vi "SubVI_PupilDetection_COLSxROWS.vi"(0 "arr":u8[][](array[numeric]), 1 "AT":u8, 2 "GB":u8, 3 "N_pts":u8, 4 "img_rows":u16=1024, 5 "img_cols":u16=1280) -> (14 "Pup_x":i16, 15 "Pup_y":i16, 16 "Radius":i16, 17 "Radius_STD":i16, 19 "error out":errorcluster)   [LabVIEW 2018]
uses:
  Pupil_cpp_dll_for_LV.dll
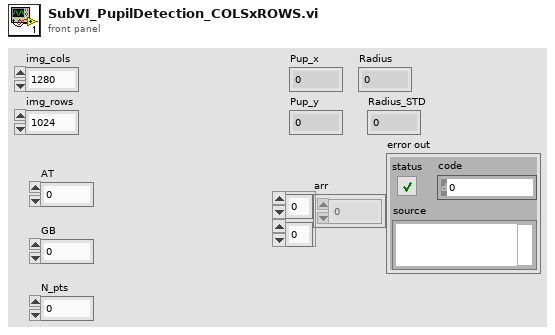
[diagram p1: front panel]
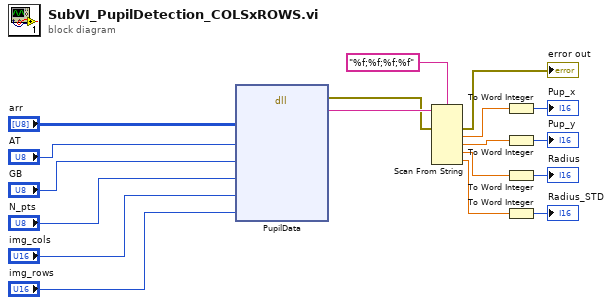
[diagram p0: block diagram]
diagram:
  n1 = dll-call lib="D:/Program_v3.0/dll/Pupil_cpp_dll_for_LV.dll" fn="PupilData"("arr"="arr", "AT"="AT", "GB"="GB", "N_pts"="N_pts", "img_cols"="img_cols", "img_rows"="img_rows") -> (error out=w2:errorcluster, "C_pupil_data"=w17:string)  [unwired: 9 in, 1 out]
  n2 = Scan From String(format string="%f;%f;%f;%f", input string=w17, error in=w2) -> (error out=→"error out":errorcluster, output 1=w14:dbl, output 2=w13:dbl, output 3=w12:dbl, output 4=w11:dbl)  [unwired: 5 in, 2 out]
  n3 = To Word Integer(number=w14) -> (16bit integer=→"Pup_x":i16)
  n4 = To Word Integer(number=w13) -> (16bit integer=→"Pup_y":i16)
  n5 = To Word Integer(number=w12) -> (16bit integer=→"Radius":i16)
  n6 = To Word Integer(number=w11) -> (16bit integer=→"Radius_STD":i16)
